vi "ParseNextStep.vi"(8 "error in (no error)":errorcluster, 9 "Result":T4, 10 "Index":T6, 11 "Qbus in":refnum<class "Qbus.lvclass">) -> (0 "error out":errorcluster)   [LabVIEW 2016, in "SeqProcessor.lvlib"]
uses:
  SeqProcessor.lvlib
  <vilib>/addons/Qbus/Qbus.lvclass
  controls/StepIndex.ctl
  controls/StepResult.ctl
  controls/StepStatus.ctl
  controls/ConditionalStep.ctl
  controls/StepAction.ctl
  controls/StepType.ctl
  controls/ParallelStep.ctl
  controls/NormalStep.ctl
  controls/JumpStep.ctl
panel:
  out "Type":T1
  out "data":T2={"Action"={"Action"="", "Process"="", "Data"=variant, "Condition"=variant(bool FALSE)}, "Result"={"Status"=enum."Undone", "Message"="", "Data"=variant}}
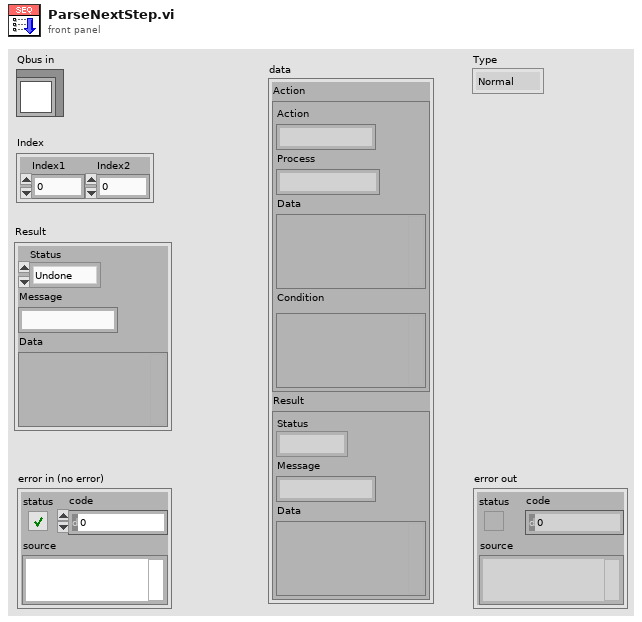
[diagram p1: front panel]
types:
  T1 = typedef "SeqProcessor.lvlib/StepType.ctl" = enum16{"Normal", "Parallel", "Conditional", "Jump"}
  T2 = typedef "SeqProcessor.lvlib/ConditionalStep.ctl" = cluster{"Action":T3, "Result":T4}
  T3 = typedef "SeqProcessor.lvlib/StepAction.ctl" = cluster{"Action":string, "Process":string, "Data":variant, "Condition":variant}
  T4 = typedef "SeqProcessor.lvlib/StepResult.ctl" = cluster{"Status":T5, "Message":string, "Data":variant}
  T5 = typedef "SeqProcessor.lvlib/StepStatus.ctl" = enum16{"Undone", "Finish", "Error"}
  T6 = typedef "SeqProcessor.lvlib/StepIndex.ctl" = cluster{"Index1":u32, "Index2":u32}
  T7 = typedef "SeqProcessor.lvlib/ParallelStep.ctl" = T8[]
  T8 = typedef "SeqProcessor.lvlib/NormalStep.ctl" = cluster{"Action":T3, "Result":T4}
  T9 = typedef "SeqProcessor.lvlib/JumpStep.ctl" = cluster{"Action":T3, "Jump":i32, "Result":T4}
  T10 = typedef "SeqProcessor.lvlib/Step.ctl" = cluster{"Type":T1, "Step":variant}
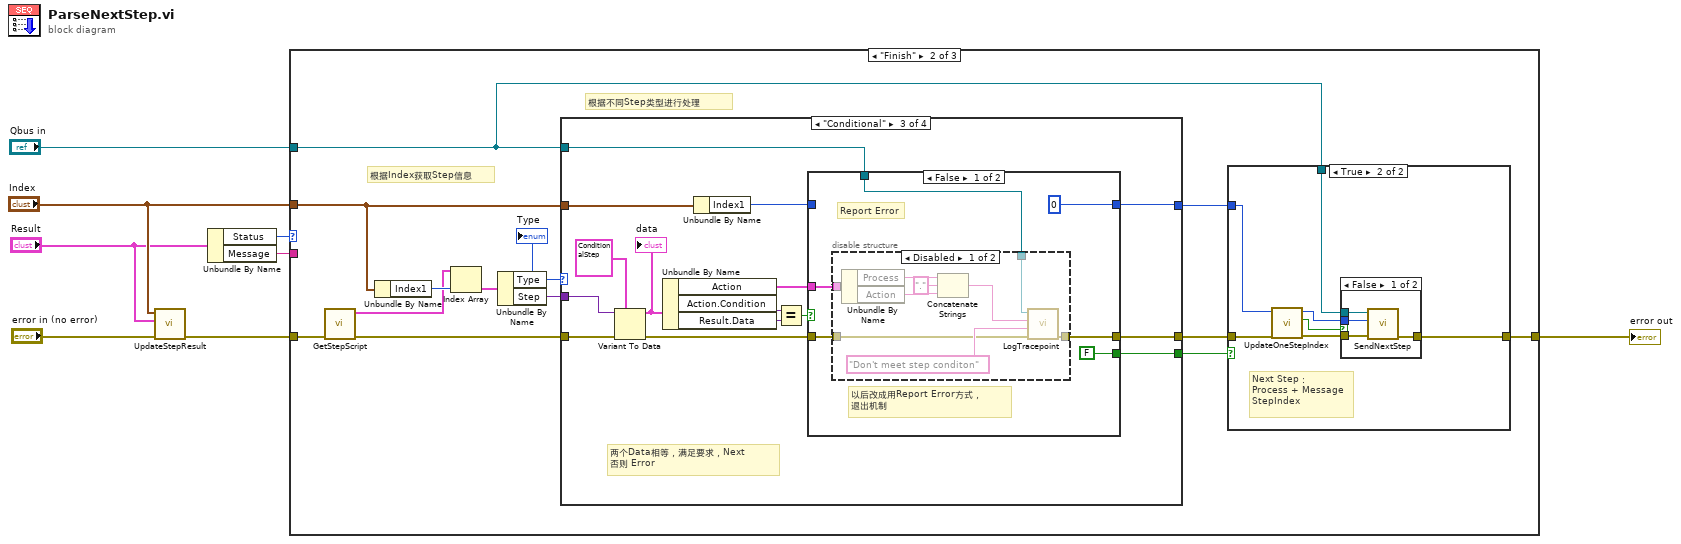
[diagram p0: block diagram]
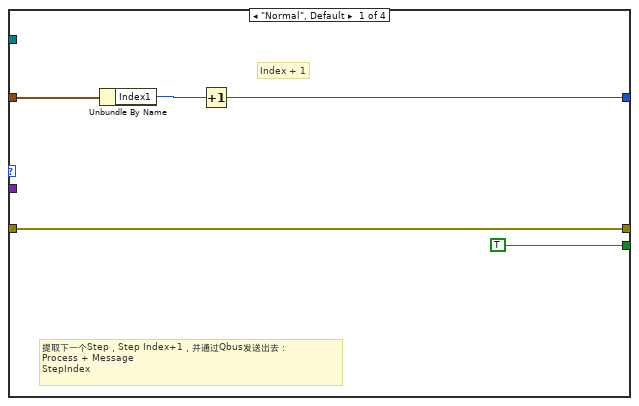
[diagram p5: hidden frame]
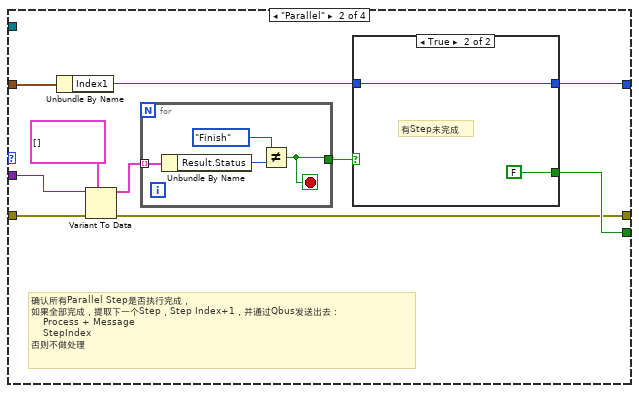
[diagram p6: hidden frame]
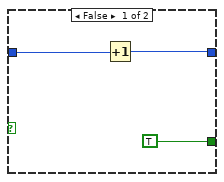
[diagram p7: hidden frame]
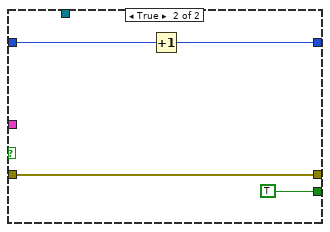
[diagram p9: hidden frame]
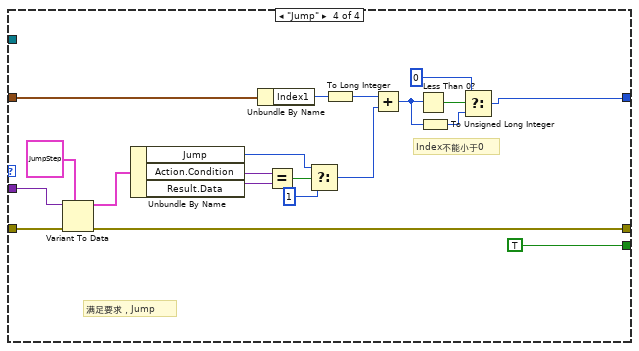
[diagram p10: hidden frame]
diagram:
  n1 = call "UpdateStepResult.vi"("error in (no error)"="error in (no error)", "Result"="Result", "Index"="Index") -> ("error out"=w5:errorcluster)  [unwired: 7 in, 1 out]
  n2 = Unbundle By Name("Result") -> ("Status"=w8:T5, "Message"=w7:string)
  n3 = case shown="\"Finish\"" w8 {
    tunnel: w7 -> [_ _ _]
    tunnel: w5 -> [w9 w18 w114]
    tunnel: "Index" -> [_ w14 _]
    tunnel: "Qbus in" -> [_ w13 _]
    tunnel: [w9 w10 w114] -> w1
    frame "Error", Default {
      # "Step出现错误，Seq直接停止，进入错误处理状态"
    }
    frame "Finish" {
      # "根据Index获取Step信息"
      # "根据不同Step类型进行处理"
      n4 = call "GetStepScript.vi"("error in (no error)"=w18) -> ("error out"=w15:errorcluster, "StepScript"=w20:T10[])  [unwired: 8 in, 1 out]
      n5 = Unbundle By Name(w14) -> ("Index1"=w21:u32)
      n6 = Index Array(array=w20, index=w21) -> (element=w17:T10)
      n7 = Unbundle By Name(w17) -> ("Type"=w19:T1, "Step"=w16:variant)
      "Type" <- w19
      n8 = case shown="\"Conditional\"" w19 {
        tunnel: [TRUE w42 w70 TRUE] -> w22
        tunnel: w14 -> [w39 w45 w74 w113]
        tunnel: w16 -> [_ w50 w73 w112]
        tunnel: w15 -> [w36 w49 w72 w111]
        tunnel: [w37 w43 w66 w99] -> w11
        tunnel: w13 -> [_ _ w65 _]
        tunnel: [w36 w41 w62 w95] -> w12
        frame "Normal", Default {
          # "Index + 1"
          # "提取下一个Step，Step Index+1，并通过Qbus发送出去：\nProcess + Message\nStepIndex"
          n9 = Unbundle By Name(w39) -> ("Index1"=w38:u32)
          n10 = Increment(x=w38) -> (x+1=w37:u32)
        }
        frame "Parallel" {
          # "确认所有Parallel Step是否执行完成，\n如果全部完成，提取下一个Step，Step Index+1，并通过Qbus发送出去：\n    Process + Message\n    StepIndex\n否则不做处理"
          n11 = Unbundle By Name(w45) -> ("Index1"=w44:u32)
          n12 = Variant To Data(error in=w49, type=T7 [] ("ParallelStep"), Variant=w50) -> (data=w47:T7, error out=w41:errorcluster)
          n13 = for {
            tunnel: w47 -> [w59] mode=indexing
            tunnel: [w56] -> w46
            stop <- w56 stop-if-true
            n14 = Unbundle By Name(w59) -> ("Result.Status"=w58:T5)
            n15 = Not Equal?(x=StepStatus."Finish" ("Result.Status"), y=w58) -> (x != y?=w56:bool)
          }
          n16 = case shown="True" w46 {
            tunnel: w44 -> [w53 w55]
            tunnel: [w52 w55] -> w43
            tunnel: [TRUE FALSE] -> w42
            frame False {
              n17 = Increment(x=w53) -> (x+1=w52:u32)
            }
            frame True {
              # "有Step未完成"
            }
          }
        }
        frame "Conditional" {
          # "两个Data相等，满足要求，Next\n否则 Error"
          n18 = Variant To Data(error in=w72, type=T2 {"Action"={"Action"="", "Process"="", "Data"=variant, "Condition"=variant(bool FALSE)}, "Result"={"Status"=enum."Undone", "Message"="", "Data"=variant}} ("ConditionlStep"), Variant=w73) -> (data=w71:T2, error out=w64:errorcluster)
          "data" <- w71
          n19 = Unbundle By Name(w71) -> ("Action"=w63:T3, "Action.Condition"=w61:variant, "Result.Data"=w60:variant)
          n20 = Unbundle By Name(w74) -> ("Index1"=w67:u32)
          n21 = Equal?(x=w61, y=w60) -> (x = y?=w68:bool)
          n22 = case shown="False" w68 {
            tunnel: [FALSE TRUE] -> w70
            tunnel: w67 -> [_ w92]
            tunnel: [u32 0 w91] -> w66
            tunnel: w65 -> [w77 _]
            tunnel: w64 -> [w76 w90]
            tunnel: w63 -> [w78 _]
            tunnel: [w75 w90] -> w62
            frame False {
              # "以后改成用Report Error方式，\n退出机制"
              # "Report Error"
              n23 = disable-structure shown="Disabled" {
                disable-tunnel: w78 -> [w89 _]
                disable-tunnel: w77 -> [w85 _]
                disable-tunnel: w76 -> [w82 _]
                disable-tunnel: [w81 _] -> w75
                frame Disabled {
                  n24 = Unbundle By Name(w89) -> ("Process"=w88:string, "Action"=w86:string)
                  n25 = Concatenate Strings(w88, "." ("string"), w86) -> (w84:string)
                  n26 = call "LogTracepoint.vi"("error in (no error)"=w82, "log string"="Don't meet step conditon", "tracepoint"=w84, "qbus in"=w85) -> ("error out"=w81:errorcluster)  [unwired: 6 in, 1 out]
                }
                frame Enabled {
                }
              }
            }
            frame True {
              n27 = Increment(x=w92) -> (x+1=w91:u32)
            }
          }
        }
        frame "Jump" {
          # "Index不能小于0"
          # "满足要求，Jump"
          n28 = Variant To Data(error in=w111, type=T9 {"Action"={"Action"="", "Process"="", "Data"=variant, "Condition"=variant(bool FALSE)}, "Jump"=0, "Result"={"Status"=enum."Undone", "Message"="", "Data"=variant}} ("JumplStep"), Variant=w112) -> (data=w110:T9, error out=w95:errorcluster)
          n29 = Unbundle By Name(w110) -> ("Jump"=w96:i32, "Action.Condition"=w109:variant, "Result.Data"=w108:variant)
          n30 = Unbundle By Name(w113) -> ("Index1"=w106:u32)
          n31 = Equal?(x=w109, y=w108) -> (x = y?=w94:bool)
          n32 = Select(t=w96, s=w94, f=1) -> (s? t:f=w105:i32)
          n33 = To Long Integer(number=w106) -> (32bit integer=w103:i32)
          n34 = Add(x=w103, y=w105) -> (x+y=w101:i32)
          n35 = Less Than 0?(x=w101) -> (x < 0?=w102:bool)
          n36 = To Unsigned Long Integer(number=w101) -> (unsigned 32bit integer=w98:u32)
          n37 = Select(t=u32 0, s=w102, f=w98) -> (s? t:f=w99:u32)
        }
      }
      n38 = case shown="True" w22 {
        tunnel: w13 -> [_ w30]
        tunnel: w12 -> [w23 w28]
        tunnel: w11 -> [_ w26]
        tunnel: [w23 w29] -> w10
        frame False {
        }
        frame True {
          # "Next Step：\nProcess + Message\nStepIndex"
          n39 = call "UpdateOneStepIndex.vi"("error in (no error)"=w28, "StepIndexIn"=w26) -> ("error out"=w27:errorcluster, "OneStep?"=w24:bool, "OneStepOut"=w25:u32)  [unwired: 7 in]
          n40 = case shown="False" w24 {
            tunnel: w30 -> [w34 _]
            tunnel: [w33 w35] -> w29
            tunnel: w27 -> [w32 w35]
            tunnel: w25 -> [w31 _]
            frame False {
              n41 = call "SendNextStep.vi"("error in (no error)"=w32, "StepIndex"=w31, "Qbus in"=w34) -> ("error out"=w33:errorcluster)  [unwired: 8 in]
            }
            frame True {
            }
          }
        }
      }
    }
    frame "Undone" {
      # "Undone，未定义，暂时不做处理"
    }
  }
  "error out" <- w1
